vi "Write Single Calibration Curve to Instrument.vi"(8 "error in (no error)":errorcluster, 9 "Channel":i32, 10 "Calibration File":path, 11 "LS218 in":refnum<class "LS218.lvclass">) -> (0 "error out":errorcluster, 3 "LS218 out":refnum<class "LS218.lvclass">)   [LabVIEW 2016, in "LS218.lvlib" / "LS218.lvclass"]
doc: "Read one calibration curve from file and write to instrument (user calibration 21-28)."
uses:
  LS218.lvclass
  C:/User/Brand/LVP/STF/Packages/CSPP_Core/Actors/CS++BaseActor/CS++BaseActor.lvclass
  CSPP_Core/Actors/CS++BaseActor/CS++BaseActor.lvclass/CS++BaseActor.ctl
  LS218.lvclass/LS218.ctl
  <vilib>/Utility/config.llb/Write Key (String).vi
  <instrlib>/Lake Shore Cryotronics 218/Lake Shore Cryotronics 218.lvlib
  <vilib>/Utility/config.llb/NI_LVConfig.lvlib
  CSPP_Core/Actors/CS++BaseActor/CS++BaseActor.lvclass
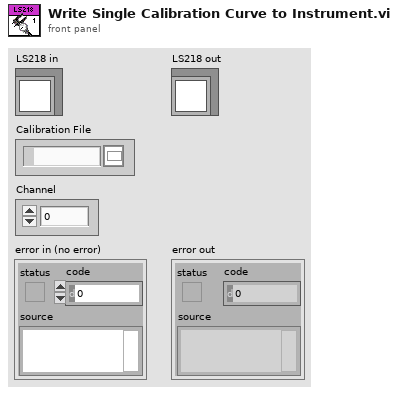
[diagram p1: front panel]
types:
  T1 = cluster{"Index (1)":i32, "Units":dbl, "Temperature":dbl}[]
  T2 = typedef "NI_LVConfig.lvlib/Config Data RefNum.ctl" = refnum<k1>
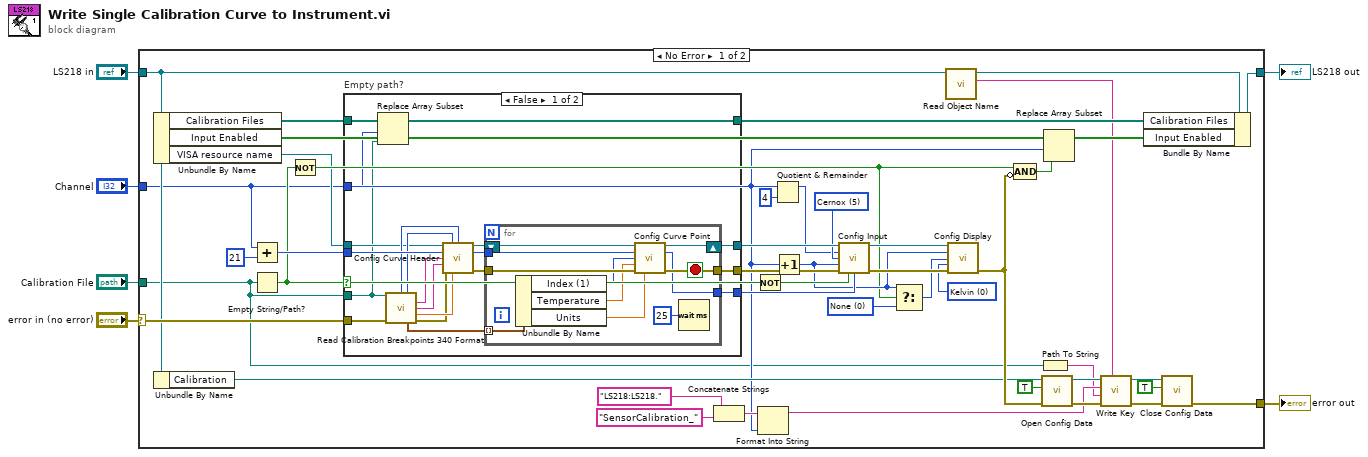
[diagram p0: block diagram]
diagram:
  n1 = case shown="No Error" "error in (no error)" {
    selector: "error in (no error)" -> [w50 w85]
    tunnel: [w8 w85] -> w5
    tunnel: [w49 w84] -> w3
    tunnel: "LS218 in" -> [w20 w84]
    tunnel: "Calibration File" -> [w13 _]
    tunnel: "Channel" -> [w15 _]
    frame No Error {
      w33 = u16 0 items=["None", "1", "2", "3", "4", "5", "6", "7", "8"] ("Input to Display(1:1)")
      w36 = u16 0 items=["Kelvin", "Celsius", "Sensor Units", "Linear Data", "Min Data", "Max Data"] ("Source (0:Kelvin)")
      w44 = u16 5 items=["2.5V Diode", "7.5V Diode", "250 Ohm Platinum", "500 Ohm Platinum", "5K Ohm Platinum", "Cernox"] ("Sensor Type (0:2.5V Diode)")
      n2 = Unbundle By Name(w20) -> ("Calibration Files"=w27:path[], "Input Enabled"=w31:bool[], "VISA resource name"=w28:refnum<visa-resource-name>)
      n3 = Unbundle By Name(w20) -> ("Calibration"=w24:path)
      n4 = Add(x=w15, y=21 ("Curve (21)")) -> (x+y=w47:i32)
      n5 = Empty String/Path?(string/path=w13) -> (empty?=w39:bool)
      n6 = Not(x=w39) -> (.not. x?=w32:bool)
      n7 = case "Empty path?" shown="False" w39 {
        tunnel: w28 -> [w53 w83]
        tunnel: w47 -> [w69 w81]
        tunnel: w50 -> [w68 w82]
        tunnel: w13 -> [w52 _]
        tunnel: [w58 w82] -> w46
        tunnel: [w57 w83] -> w45
        tunnel: [w56 w81] -> w43
        tunnel: w27 -> [w55 w80]
        tunnel: w15 -> [w54 _]
        tunnel: [w51 w80] -> w26
        frame False {
          n8 = Replace Array Subset(array=w55, new element=w52, index=w54) -> (w51:path[])
          n9 = call "Read Calibration Breakpoints 340 Format.vi"("Calibration File"=w52, "Error In"=w68) -> ("Temp Coefficient"=w62:u16, "Curve Data Format"=w63:u16, "Curve Name"=w65:string, "Curve Serial Number"=w64:string, "Limit Value"=w61:dbl, "Calibration Points"=w59:T1, "Error Out"=w60:errorcluster)  [unwired: 7 in]
          n10 = call <instrlib>:"Config Curve Header.vi"("VISA resource name"=w53, "Curve Data Format (V/K:0)"=w63, "Temp Coefficient (Neg:0)"=w62, "Curve (21)"=w69, "Curve Name (\"\")"=w65, "Curve Serial Number (\"\")"=w64, "error in (no error)"=w60, "Limit Value (475.00)"=w61) -> ("VISA resource name out"=w67:refnum<visa-resource-name>, "error out"=w66:errorcluster)  [unwired: 6 in]
          n11 = for {
            tunnel: w69 -> [w70]
            tunnel: w59 -> [w76] mode=indexing
            tunnel: w66 -> [w78]
            tunnel: [w77] -> w58
            tunnel: [w70] -> w56
            shift-right: [w71] -> w57
            shift-left: w67 -> [w79]
            stop <- w77 stop-if-true
            n12 = Unbundle By Name(w76) -> ("Index (1)"=w75:i32, "Temperature"=w74:dbl, "Units"=w73:dbl)
            n13 = call <instrlib>:"Config Curve Point.vi"("VISA resource name"=w79, "Units Value (0.0000)"=w73, "Curve (21)"=w70, "Index (1)"=w75, "Temperature Value (0.0000)"=w74, "error in (no error)"=w78) -> ("VISA resource name out"=w71:refnum<visa-resource-name>, "error out"=w77:errorcluster)  [unwired: 8 in]
            n14 = Wait (ms)(milliseconds to wait=u32 25) -> ()  [unwired: 1 out]
          }
        }
        frame True {
          # "#Todo Make calibration invalid"
        }
      }
      n15 = Concatenate Strings("LS218:LS218.", "SensorCalibration_" ("string")) -> (w16:string)
      n16 = Not(x=w39) -> (.not. x?=w40:bool)
      n17 = Format Into String(initial string=w16, w15) -> (resulting string=w14:string)  [unwired: 2 in, 1 out]
      n18 = Quotient & Remainder(x=w15, y=4) -> (x-y*floor(x/y)=w42:i32)  [unwired: 1 out]
      n19 = Increment(x=w15) -> (x+1=w35:i32)
      n20 = call <instrlib>:"Config Input.vi"("VISA resource name"=w45, "Input Group (0:Inputs 1-4)"=w42, "Sensor Type (0:2.5V Diode)"=w44, "Input (1)"=w35, "error in (no error)"=w46, "Input (T: Input ON)"=w40, "Input Curve (0:None)"=w43) -> ("VISA resource name out"=w38:refnum<visa-resource-name>, "error out"=w37:errorcluster)  [unwired: 7 in]
      n21 = Select(t=w35, s=w32, f=w33) -> (s? t:f=w34:i32)
      n22 = call "Read Object Name.vi"("CS++BaseActor in"=w20) -> ("Object Name"=w12:string, "CS++BaseActor out"=w19:refnum<class "LS218.lvclass">)  [unwired: 8 in, 1 out]
      n23 = call <instrlib>:"Config Display.vi"("VISA resource name"=w38, "Display Field (1)"=w35, "Input to Display(1:1)"=w34, "Source (0:Kelvin)"=w36, "error in (no error)"=w37) -> ("error out"=w25:errorcluster)  [unwired: 9 in, 1 out]
      n24 = Compound Arithmetic op=AND(w32, invert w25) -> (w29:bool)
      n25 = Path To String(path=w13) -> (string=w7:string)
      n26 = call <vilib>:"Open Config Data.vi"("error in (no error)"=w25, "create file if necessary (T)"=TRUE, "configuration file path"=w24) -> ("error out"=w21:errorcluster, "refnum"=w22:T2)  [unwired: 6 in, 1 out]
      n27 = Replace Array Subset(array=w31, new element=w29, index=w15) -> (w30:bool[])
      n28 = call-poly <vilib>:"Write Key.vi"("section"=w12, "error in (no error)"=w21, "value"=w7, "key"=w14, "refnum"=w22) -> ("error out"=w11:errorcluster, "refnum out"=w10:T2)  [unwired: 4 in, 1 out]
      n29 = Bundle By Name(cluster=w19, "Calibration Files"=w26, "Input Enabled"=w30) -> (w49:refnum<class "LS218.lvclass">)
      n30 = call <vilib>:"Close Config Data.vi"("error in (no error)"=w11, "write file if changed (T)"=TRUE, "refnum"=w10) -> ("error out"=w8:errorcluster)  [unwired: 7 in, 1 out]
    }
    frame Error {
    }
  }
  "error out" <- w5
  "LS218 out" <- w3
